vi "Attach Observer.vi"(8 "error in":errorcluster, 10 "Subject":i32, 11 "GUI Facade in":refnum<class "GUI Facade.lvclass">) -> (0 "error out":errorcluster, 2 "Observer":refnum<queue>, 3 "GUI Facade out":refnum<class "GUI Facade.lvclass">)   [LabVIEW 2018, in "GUI Facade.lvclass"]
doc: "Attach an observer to a subject that is not necessarily related to a UI (i.e. file writing, process monitoring, etc)."
uses:
  GUI Facade.lvclass
  Observer/Data Subject.lvclass
  Data/Data.lvclass
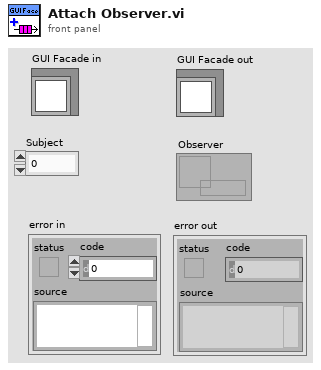
[diagram p1: front panel]
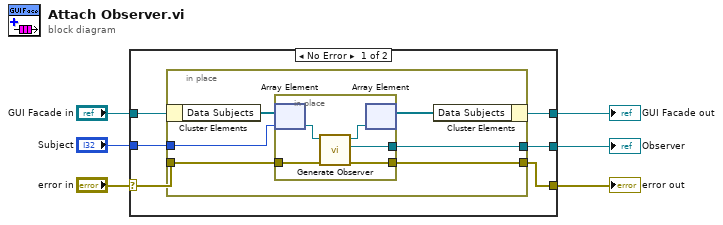
[diagram p0: block diagram]
diagram:
  n1 = case shown="No Error" "error in" {
    selector: "error in" -> [w11 w25]
    tunnel: [w10 w25] -> w5
    tunnel: [w8 w24] -> w3
    tunnel: "GUI Facade in" -> [w9 w24]
    tunnel: "Subject" -> [w12 _]
    tunnel: [w7 _] -> w1
    frame No Error {
      n2 = in-place {
        in-place-border: w12 -> [w17]
        in-place-border: w11 -> [w16]
        in-place-border: [w15] -> w10
        in-place-border: [w14] -> w7
        n3 = in-place-cluster #1(w9) -> ("Data Subjects"=w18:refnum<class "Data Subject.lvclass">[])
        n4 = in-place {
          in-place-border: w16 -> [w23]
          in-place-border: [w22] -> w15
          in-place-border: [w19] -> w14
          n5 = in-place-array #2(w18, w17) -> (w21:refnum<class "Data Subject.lvclass">)
          n6 = call "Generate Observer.vi"("error in"=w23, "Data Subject in"=w21) -> ("error out"=w22:errorcluster, "Observer"=w19:refnum<queue>, "Data Subject out"=w20:refnum<class "Data Subject.lvclass">)  [unwired: 7 in]
          n7 = in-place-array #2(w20) -> (w13:refnum<class "Data Subject.lvclass">[])  [unwired: 1 out]
        }
        n8 = in-place-cluster #1("Data Subjects"=w13) -> (w8:refnum<class "GUI Facade.lvclass">)
      }
    }
    frame Error {
    }
  }
  "error out" <- w5
  "GUI Facade out" <- w3
  "Observer" <- w1
